vi "Objects to Configurations.vi"(8 "error in (no error)":errorcluster, 11 "Objects in":T1) -> (0 "error out":errorcluster, 1 "engine configuration out":refnum<class "engine configuration.lvclass">, 2 "tag bus configurable plugin module configuration":refnum<class "Multiplexer configuration.lvclass">)   [LabVIEW 2021, in "Multiplexer editor node.lvclass"]
doc: "This VI gets the configurations from the objects references. This VI is moslty used for Read only operations."
uses:
  Multiplexer editor node.lvclass
  configuration/Multiplexer configuration.lvclass
  <vilib>/NI/Module Execution Interface/Engine Configuration/engine configuration.lvclass
  <vilib>/NI/DCAF/Tag Editor Core/Table API/Table Manager/object ref.ctl
  <vilib>/NI/DCAF/Tag Editor Core/Configuration Editor/Classes/Engine Parent/Engine Parent Editor Node.lvclass
  C:/Program Files (x86)/National Instruments/LabVIEW 2021/vi.lib/NI/Configuration Framework/serializable node/NISE_CEF_serializable node.lvclass
  <vilib>/NI/DCAF/Tag Editor Core/Configuration Editor/Classes/Module editor node/module editor node.lvclass
  <vilib>/NI/Configuration Framework/serializable configuration/NISE_CEF_serializable configuration.lvclass
  Multiplexer editor node.lvclass/Multiplexer editor node.ctl
  <vilib>/NI/DCAF/Tag Editor Core/Table API/Table Manager/Table Manager.lvclass
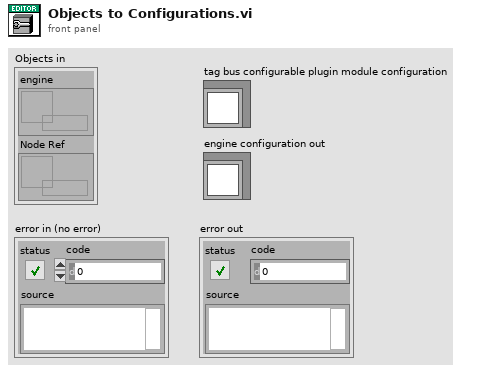
[diagram p1: front panel]
types:
  T1 = typedef "Table Manager.lvlib/Table Manager.lvclass/object ref.ctl" = cluster{"engine":refnum<data-value>, "Node Ref":refnum<data-value>}
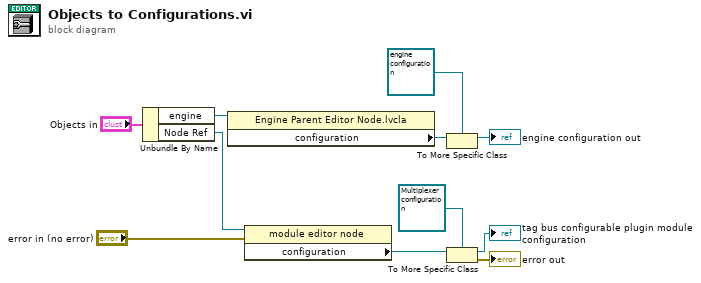
[diagram p0: block diagram]
diagram:
  n1 = Unbundle By Name("Objects in") -> ("engine"=w2:refnum<data-value>, "Node Ref"=w6:refnum<data-value>)
  n2 = property class="Engine Parent Editor Node.lvcla"(reference=w2) -> ("configuration"=w4:refnum<class "NISE_CEF_serializable configuration.lvclass">)  [unwired: 1 in, 2 out]
  n3 = property class="module editor node"(reference=w6, error in="error in (no error)") -> ("configuration"=w7:refnum<class "NISE_CEF_serializable configuration.lvclass">)  [unwired: 2 out]
  n4 = To More Specific Class(target class=refnum<class "engine configuration.lvclass"> refnum ("engine configuration out"), reference=w4) -> (specific class reference=→"engine configuration out":refnum<class "engine configuration.lvclass">)  [unwired: 1 in, 1 out]
  n5 = To More Specific Class(target class=refnum<class "Multiplexer configuration.lvclass"> refnum ("tag bus configurable plugin module configuration"), reference=w7) -> (specific class reference=→"tag bus configurable plugin module configuration":refnum<class "Multiplexer configuration.lvclass">, error out=→"error out":errorcluster)  [unwired: 1 in]
